vi "generazione rivelatore.vi"(8 "error in":errorcluster) -> (0 "error out":errorcluster, 3 "Detector Out":dbl[][](array[numeric]))   [LabVIEW 2023]
uses:
  <vilib>/Utility/file.llb/Read Delimited Spreadsheet (DBL).vi
  <vilib>/Utility/file.llb/Write Delimited Spreadsheet (DBL).vi
panel:
  in  "Save":bool
  in  "Transpose File?":bool=TRUE
  in  "Number Bin":dbl
  in  "norm":bool
  in  "bin":bool
  out "XY Graph":cluster{"all rows":dbl[], "all rows":dbl[]}(graph)
  in  "Stop":bool
  in  "List Detectors":string(combo)
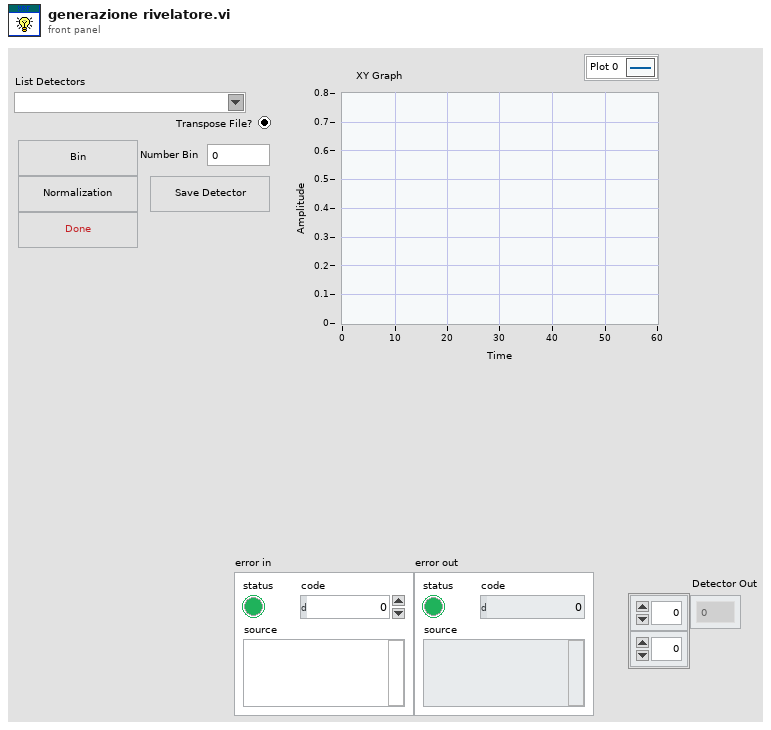
[diagram p1: front panel]
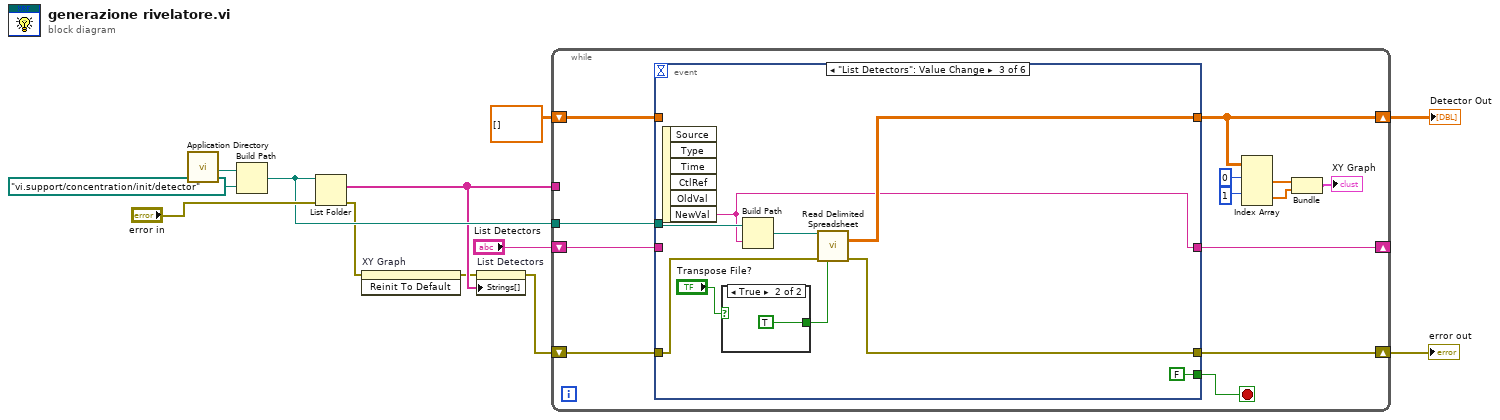
[diagram p0: block diagram]
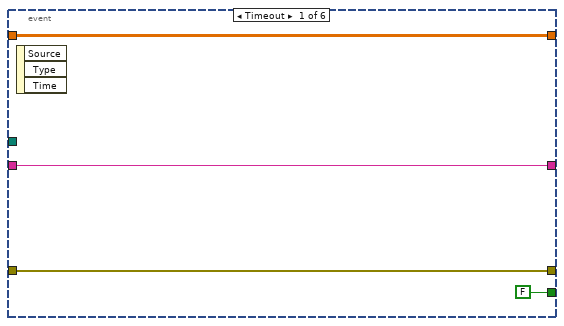
[diagram p2: hidden frame]
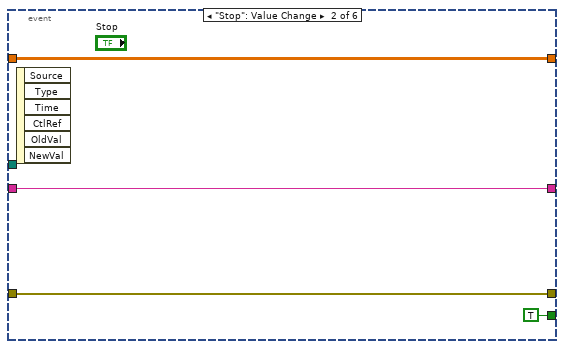
[diagram p3: hidden frame]
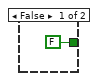
[diagram p4: hidden frame]
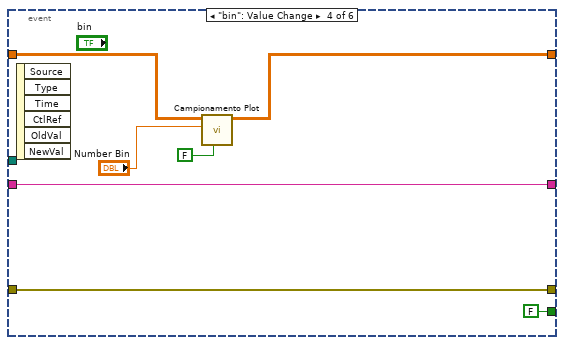
[diagram p5: hidden frame]
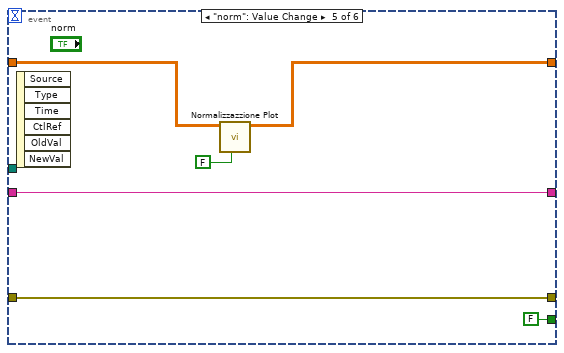
[diagram p6: hidden frame]
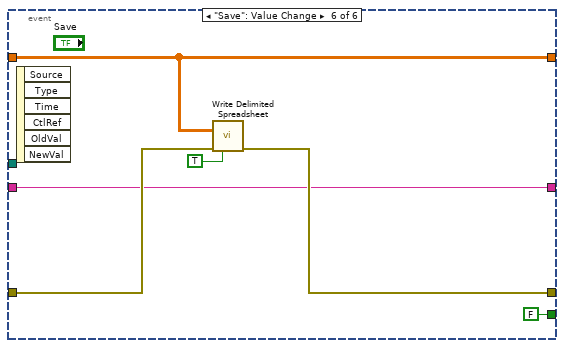
[diagram p7: hidden frame]
diagram:
  n1 = call <vilib>:"Application Directory.vi"() -> ("Application Directory"=w12:path)
  n2 = Build Path(base path=w12, name or relative path=path "vi.support/concentration/init/detector") -> (appended path=w7:path)
  n3 = List Folder(path=w7, error in="error in") -> (filenames=w6:string[], error out=w3:errorcluster)  [unwired: 2 in, 2 out]
  n4 = invoke on="XY Graph" class="XYGraph (strict)" method="Reinit To Default"(error in=w3) -> (error out=w2:errorcluster)  [unwired: 2 in, 2 out]
  n5 = property on="List Detectors" class="CmbBox"(error in=w2, "Strings[]"=w6) -> (error out=w5:errorcluster)  [unwired: 1 in, 1 out]
  n6 = while {
    tunnel: w6 -> [_]
    shift-right: [w24] -> w9
    shift-left: w5 -> [w23]
    shift-right: [w21] -> _
    shift-left: "List Detectors" -> [w22]
    tunnel: w7 -> [w20]
    shift-right: [w15] -> w1
    shift-left: dbl[][] [] ("all rows") -> [w19]
    stop <- w25 stop-if-true
    n7 = event shown="[2] \"List Detectors\": Value Change" {
      selector: _ -> [_ _ _ _ _ _]
      dyn-events: _ -> [_ _ _ _ _ _]
      timeout: _ -> [_ _ _ _ _ _]
      tunnel: [FALSE TRUE FALSE FALSE FALSE FALSE] -> w25
      tunnel: [w28 w32 w39 w47 w56 w59] -> w24
      tunnel: w23 -> [w28 w32 w40 w47 w56 w60]
      tunnel: w22 -> [w27 w31 _ w46 w55 w58]
      tunnel: [w27 w31 w34 w46 w55 w58] -> w21
      tunnel: w20 -> [_ _ w42 _ _ _]
      tunnel: [w26 w30 w37 w48 w52 w62] -> w15
      tunnel: w19 -> [w26 w30 _ w50 w53 w62]
      event Timeout {
        n8 = event-data() -> ()  [unwired: 1 in, 3 out]
      }
      event "Stop": Value Change {
        n9 = event-data() -> ()  [unwired: 1 in, 6 out]
      }
      event "List Detectors": Value Change {
        n10 = event-data() -> ("NewVal"=w34:string)  [unwired: 1 in, 5 out]
        n11 = case shown="True" "Transpose File?" {
          tunnel: [FALSE ("transpose? (F)") TRUE ("transpose? (F)")] -> w36
          frame False {
          }
          frame True {
          }
        }
        n12 = Build Path(base path=w42, name or relative path=w34) -> (appended path=w41:path)
        n13 = call-poly <vilib>:"Read Delimited Spreadsheet.vi"("file path (dialog if empty)"=w41, "error in (no error)"=w40, "transpose? (F)"=w36) -> ("all rows"=w37:dbl[][], "error out"=w39:errorcluster)  [unwired: 7 in, 4 out]
      }
      event "bin": Value Change {
        n14 = event-data() -> ()  [unwired: 1 in, 6 out]
        n15 = call "Campionamento Plot.vi"("External File?"=FALSE, "Num Max"="Number Bin", "Spectrum In"=w50) -> ("Spectrum Out"=w48:dbl[][])  [unwired: 8 in]
      }
      event "norm": Value Change {
        n16 = event-data() -> ()  [unwired: 1 in, 6 out]
        n17 = call "Normalizzazzione Plot.vi"("External File?"=FALSE, "Spectrum In"=w53) -> ("Spectrum Out"=w52:dbl[][])  [unwired: 9 in]
      }
      event "Save": Value Change {
        n18 = event-data() -> ()  [unwired: 1 in, 6 out]
        n19 = call-poly <vilib>:"Write Delimited Spreadsheet.vi"("2D data"=w62, "error in (no error)"=w60, "transpose? (no:F)"=TRUE) -> ("error out"=w59:errorcluster)  [unwired: 11 in, 1 out]
      }
    }
    n20 = Index Array(array=w15, index (row) #1=0 ("index (row)"), index (row) #2=1 ("index (row)")) -> (element #1=w16:dbl[], element #2=w17:dbl[])  [unwired: 2 in]
    n21 = Bundle("all rows"=w16, "all rows"=w17) -> (→"XY Graph":cluster{"all rows":dbl[], "all rows":dbl[]})  [unwired: 1 in]
  }
  "error out" <- w9
  "Detector Out" <- w1
